vi "Ex3.vi"() -> ()   [LabVIEW 2016]
uses:
  <vilib>/Utility/file.llb/Write Delimited Spreadsheet (string).vi
panel:
  out "테이블 컨트롤":string[][](table)
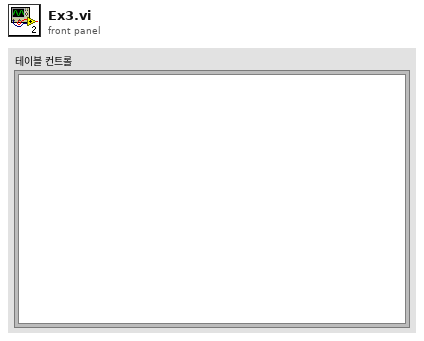
[diagram p1: front panel]
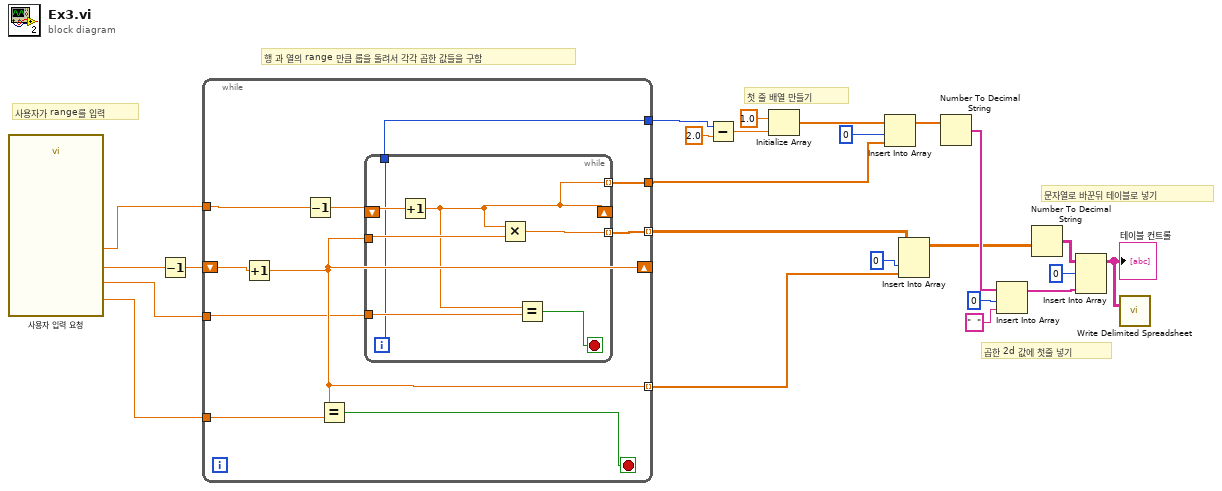
[diagram p0: block diagram]
diagram:
  # "문자열로 바꾼뒤 테이블로 넣기"
  # "행 과 열의 range 만큼 룹을 돌려서 각각 곱한 값들을 구함"
  # "사용자가 range를 입력"
  # "곱한 2d 값에 첫줄 넣기"
  # "첫 줄 배열 만들기"
  n1 = call "사용자 입력 요청"() -> ("Multiplier end point"=w11:dbl, "Multiplier start point"=w14:dbl, "Multiplicand end point"=w12:dbl, "Multiplicand start point"=w13:dbl)  [unwired: 14 in, 2 out]
  n2 = Decrement(x=w14) -> (x-1=w24:dbl)
  n3 = while {
    shift-right: [w29] -> _
    shift-left: w24 -> [w34]
    tunnel: [w32] -> w3 mode=indexing
    tunnel: [w31] -> w18
    tunnel: [w30] -> w2
    tunnel: [w29] -> w17 mode=indexing
    tunnel: w13 -> [w28]
    tunnel: w12 -> [w26]
    tunnel: w11 -> [w27]
    stop <- w25 stop-if-true
    n4 = Increment(x=w34) -> (x+1=w29:dbl)
    n5 = Decrement(x=w28) -> (x-1=w33:dbl)
    n6 = Equal?(x=w29, y=w27) -> (x = y?=w25:bool)
    n7 = while {
      tunnel: w29 -> [w39]
      shift-right: [w37] -> _
      shift-left: w33 -> [w41]
      tunnel: [w38] -> w32 mode=indexing
      tunnel: [w35] -> w31
      tunnel: [w37] -> w30 mode=indexing
      tunnel: w26 -> [w36]
      i -> [w35]
      stop <- w40 stop-if-true
      n8 = Increment(x=w41) -> (x+1=w37:dbl)
      n9 = Multiply(x=w37, y=w39) -> (x*y=w38:dbl)
      n10 = Equal?(x=w37, y=w36) -> (x = y?=w40:bool)
    }
  }
  n11 = Subtract(x=w18, y=2.0) -> (x-y=w19:dbl)
  n12 = Initialize Array(1.0 ("원소"), w19) -> (w22:dbl[])
  n13 = Insert Into Array(array=w22, index=0 ("인덱스"), new element=w2) -> (w1:dbl[])
  n14 = Insert Into Array(array=w3, index (col)=0 ("인덱스 (행)"), new element=w17) -> (w8:dbl[][])  [unwired: 1 in]
  n15 = Number To Decimal String(number=w1) -> (decimal integer string=w10:string[])  [unwired: 1 in]
  n16 = Insert Into Array(array=w10, index=0 ("인덱스"), new element="  ") -> (w6:string[])
  n17 = Number To Decimal String(number=w8) -> (decimal integer string=w7:string[][])  [unwired: 1 in]
  n18 = Insert Into Array(array=w7, index (row)=0 ("인덱스 (행)"), new element=w6) -> (w4:string[][])  [unwired: 1 in]
  "테이블 컨트롤" <- w4
  n19 = call-poly <vilib>:"Write Delimited Spreadsheet.vi"("2D data"=w4) -> ()  [unwired: 13 in, 2 out]
